vi "setRow.vi"(7 "bus":T1, 8 "error in":errorcluster) -> (0 "error out":errorcluster)   [LabVIEW 2020]
uses:
  bus.ctl
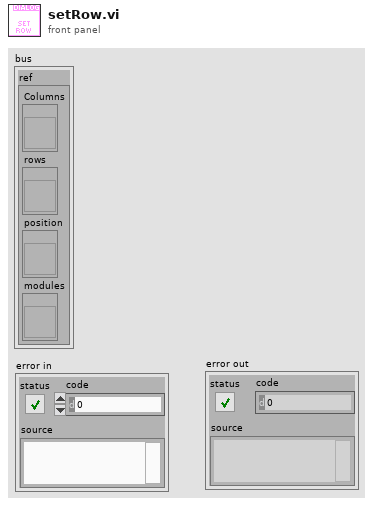
[diagram p1: front panel]
types:
  T1 = typedef "bus.ctl" = cluster{"ref":cluster{"Columns":refnum<vi>, "rows":refnum<vi>, "position":refnum<vi>, "modules":refnum<vi>}}
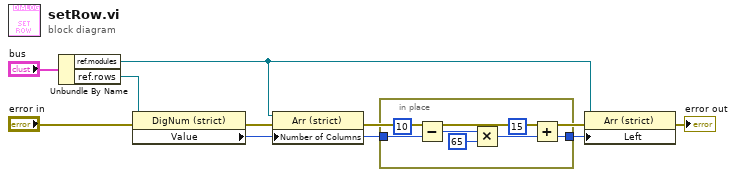
[diagram p0: block diagram]
diagram:
  n1 = Unbundle By Name("bus") -> ("ref.modules"=w5:refnum<vi>, "ref.rows"=w6:refnum<vi>)
  n2 = property class="DigNum (strict)"(reference=w6, error in="error in") -> (error out=w9:errorcluster, "Value"=w2:u8)  [unwired: 1 out]
  n3 = property on="Property Node" class="Arr (strict)"(reference=w5, error in=w9, "Number of Columns"=w2) -> (error out=w7:errorcluster)  [unwired: 1 out]
  n4 = in-place {
    in-place-border: w2 -> [w11]
    in-place-border: [w10] -> w1
    n5 = Subtract(x=10, y=w11) -> (x-y=w12:i32)
    n6 = Multiply(x=w12, y=65) -> (x*y=w14:i32)
    n7 = Add(x=15, y=w14) -> (x+y=w10:i32)
  }
  n8 = property on="Property Node" class="Arr (strict)"(reference=w5, error in=w7, "Left"=w1) -> (error out=→"error out":errorcluster)  [unwired: 1 out]
